vi "rand_ave.vi"(1 "最小值":string, 2 "最大值":string, 3 "偏移值":dbl=1.0) -> (0 "结果":string)   [LabVIEW 2011]
doc: "采用随机数法生成的最大值，最小值中间的一个数值，偏移值用来控制生成的值偏向"
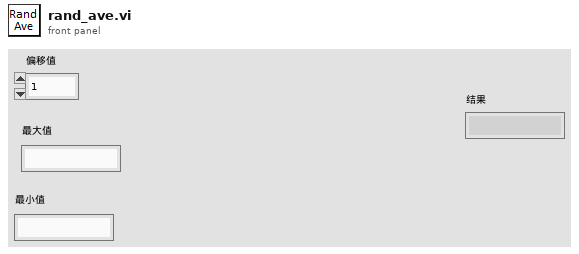
[diagram p1: front panel]
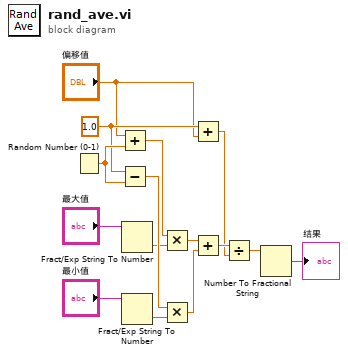
[diagram p0: block diagram]
diagram:
  w9 = 1.0 ("x")
  n1 = Random Number (0-1)() -> (number: 0 to 1=w15:dbl)
  n2 = Add(x="偏移值", y=w15) -> (x+y=w13:dbl)
  n3 = Subtract(x=w9, y=w15) -> (x-y=w14:dbl)
  n4 = Fract/Exp String To Number(string="最大值") -> (number=w3:dbl)  [unwired: 3 in, 1 out]
  n5 = Fract/Exp String To Number(string="最小值") -> (number=w1:dbl)  [unwired: 3 in, 1 out]
  n6 = Multiply(x=w13, y=w3) -> (x*y=w12:dbl)
  n7 = Multiply(x=w14, y=w1) -> (x*y=w11:dbl)
  n8 = Add(x=w9, y="偏移值") -> (x+y=w7:dbl)
  n9 = Add(x=w12, y=w11) -> (x+y=w10:dbl)
  n10 = Divide(x=w10, y=w7) -> (x/y=w6:dbl)
  n11 = Number To Fractional String(number=w6) -> (F-format string=→"结果":string)  [unwired: 3 in]
